vi "Read Multi Eval Meas ACLR Results.vi"(8 "error in (no error)":errorcluster, 9 "Result Type (Current)":i32(ring) items=["Current", "Average"], 10 "Instance (1)":T2=1, 11 "VISA resource name":refnum<visa-resource-name>) -> (0 "error out":errorcluster, 1 "ACLR Results":T1 {"NR Pos" format="%^.3e"; "Carrier" format="%^.3e"; "NR Neg" format="%^.3e"}, 2 "Reliability":i32, 3 "VISA resource name out":refnum<visa-resource-name>)   [LabVIEW 2020, in "Rohde&Schwarz CMXP NR FR2 Measurement.lvlib"]
doc: "Starts a new single shot measurement and returns the multi eval measurement ACLR results.\n\nAttributes:\nRSCMXPNRFR2M_ATTR_READ_MULTI_EVAL_MEASUREMENT_ACLR_AVERAGE_RESULTS\nRSCMXPNRFR2M_ATTR_READ_MULTI_EVAL_MEASUREMENT_ACLR_CURRENT_RESULTS\n\nRemote-control commands:\nREAD:NRMMw:MEAS<i>:MEValuation:ACLR:AVERage?\nREAD:NRMMw:MEAS<i>:MEValuation:ACLR:CURRent?"
uses:
  <instrlib>/Rohde&Schwarz CMXP NR FR2 Measurement/Rohde&Schwarz CMXP NR FR2 Measurement.lvlib
  <instrlib>/Rohde&Schwarz CMXP NR FR2 Measurement/Private/_Instance.ctl
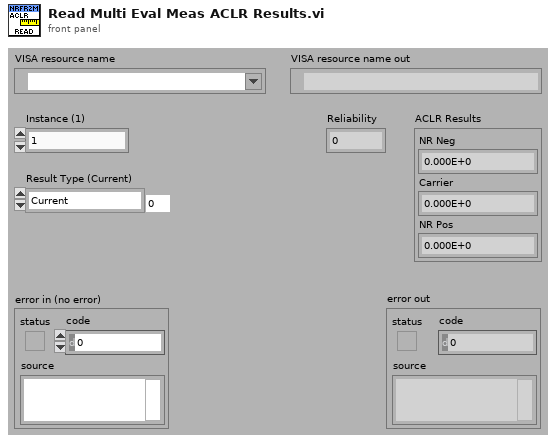
[diagram p1: front panel]
types:
  T1 = cluster{"NR Neg":dbl, "Carrier":dbl, "NR Pos":dbl}
  T2 = typedef "Rohde&Schwarz CMXP NR FR2 Measurement.lvlib/_Instance.ctl" = i32
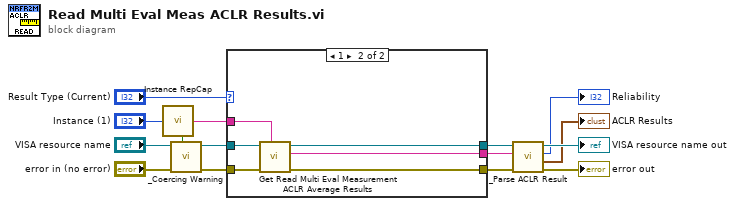
[diagram p0: block diagram]
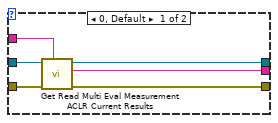
[diagram p2: hidden frame]
diagram:
  n1 = call <instrlib>:"Instance RepCap.vi"("Instance In"="Instance (1)") -> ("In Range?"=w4:bool, "RepCap Identifier Out"=w5:string)  [unwired: 1 in]
  n2 = call <instrlib>:"_Coercing Warning.vi"("In Range?"=w4, "error in (no error)"="error in (no error)", "VISA resource name"="VISA resource name") -> ("error out"=w2:errorcluster, "VISA resource name out"=w3:refnum<visa-resource-name>)  [unwired: 7 in]
  n3 = case shown="1" "Result Type (Current)" {
    tunnel: w2 -> [w20 w27]
    tunnel: w3 -> [w21 w26]
    tunnel: [w18 w25] -> w13
    tunnel: [w19 w24] -> w11
    tunnel: [w17 w23] -> w14
    tunnel: w5 -> [w16 w22]
    frame 0, Default {
      n4 = call "Get Read Multi Eval Measurement ACLR Current Results"("Repeated Capabilities"=w16, "error in (no error)"=w20, "instrument handle"=w21) -> ("error out"=w18:errorcluster, "Read Multi Eval Measurement ACLR Current Results"=w17:string, "instrument handle out"=w19:refnum<visa-resource-name>)  [unwired: 6 in]
    }
    frame 1 {
      n5 = call "Get Read Multi Eval Measurement ACLR Average Results"("Repeated Capabilities"=w22, "error in (no error)"=w27, "instrument handle"=w26) -> ("error out"=w25:errorcluster, "Read Multi Eval Measurement ACLR Average Results"=w23:string, "instrument handle out"=w24:refnum<visa-resource-name>)  [unwired: 6 in]
    }
  }
  n6 = call <instrlib>:"_Parse ACLR Result.vi"("error in (no error)"=w13, "Input String"=w14, "VISA resource name"=w11) -> ("error out"=→"error out":errorcluster, "Measurement Result"=→"ACLR Results":T1, "Reliability"=→"Reliability":i32, "VISA resource name out"=→"VISA resource name out":refnum<visa-resource-name>)  [unwired: 5 in]
